vi "Check Transfer.vi"(8 "error in":errorcluster, 10 "TransferOperationResult":refnum<k24>, 11 "FileTransfer in":refnum<class "FileTransfer.lvclass">) -> (0 "error out":errorcluster, 3 "FileTransfer out":refnum<class "FileTransfer.lvclass">)   [LabVIEW 2015, in "WinSCP.lvlib" / "FileTransfer.lvclass"]
uses:
  FileTransfer.lvclass
  C:/Program Files (x86)/WinSCP/WinSCPnet.dll
  Program Files (x86)/WinSCP/WinSCPnet.dll
panel:
  out "Array 3":cluster{"Message":string, "Source":string}[](array[cluster])
  out "Array 2":T1(array[cluster])
  out "IsSuccess":bool
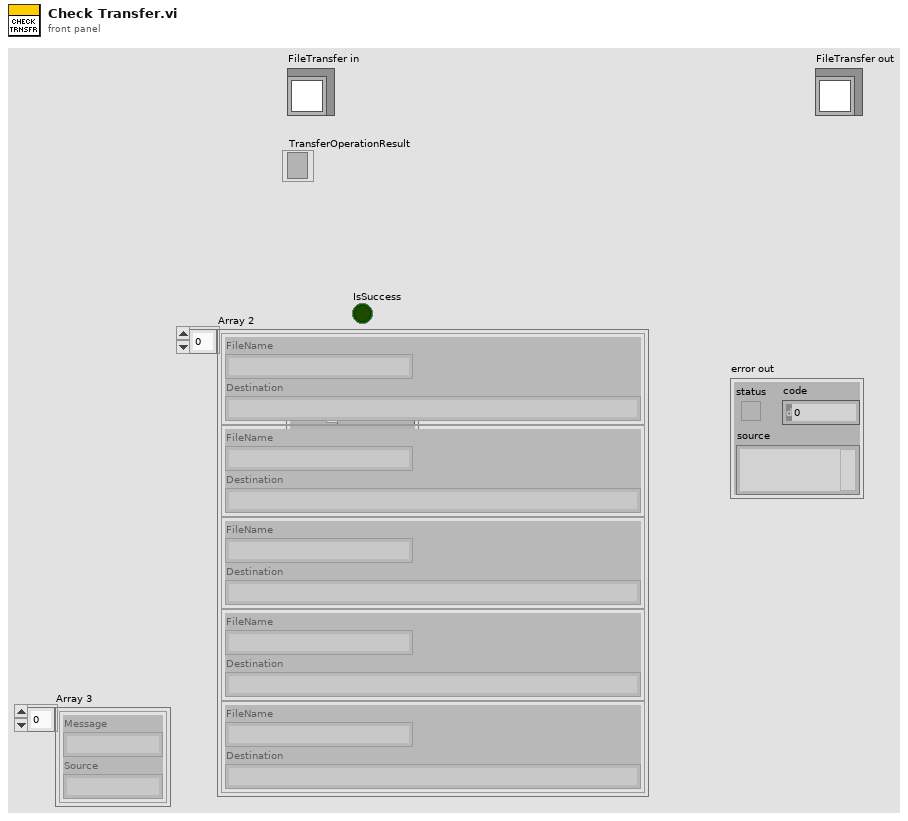
[diagram p1: front panel]
types:
  T1 = cluster{"FileName":string, "Destination":string}[]
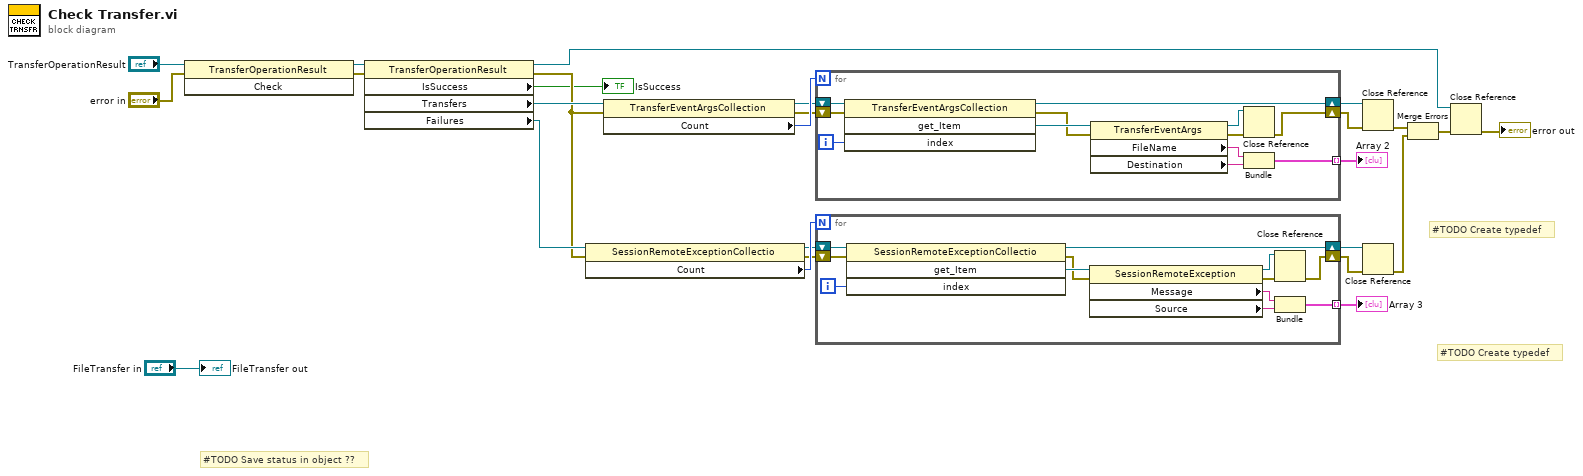
[diagram p0: block diagram]
diagram:
  # "#TODO Save status in object ??"
  # "#TODO Create typedef"
  # "#TODO Create typedef"
  n1 = invoke class="TransferOperationResult" method="Check"(reference="TransferOperationResult", error in="error in") -> (reference out=w25:refnum<k24>, error out=w8:errorcluster)  [unwired: 1 in, 1 out]
  n2 = property class="TransferOperationResult"(reference=w25, error in=w8) -> (reference out=w19:refnum<k24>, error out=w7:errorcluster, "IsSuccess"=→"IsSuccess":bool, "Transfers"=w24:refnum<k24>, "Failures"=w18:refnum<k24>)
  n3 = property class="SessionRemoteExceptionCollectio"(reference=w18, error in=w7) -> (reference out=w16:refnum<k24>, error out=w3:errorcluster, "Count"=w17:i32)
  n4 = property class="TransferEventArgsCollection"(reference=w24, error in=w7) -> (reference out=w22:refnum<k24>, error out=w5:errorcluster, "Count"=w23:i32)
  n5 = for {
    N: w23 -> [_]
    shift-right: [w33] -> w20
    shift-left: w22 -> [w38]
    tunnel: [w32] -> w21 mode=indexing
    shift-right: [w27] -> w4
    shift-left: w5 -> [w29]
    i -> [w37]
    n6 = invoke class="TransferEventArgsCollection" method="get_Item"(reference=w38, error in=w29, "index"=w37) -> (reference out=w33:refnum<k24>, error out=w28:errorcluster, "get_Item"=w36:refnum<k24>)  [unwired: 1 in, 1 out]
    n7 = property class="TransferEventArgs"(reference=w36, error in=w28) -> (reference out=w30:refnum<k24>, error out=w31:errorcluster, "FileName"=w35:string, "Destination"=w34:string)
    n8 = Close Reference(reference=w30, error in (no error)=w31) -> (error out=w27:errorcluster)
    n9 = Bundle("FileName"=w35, "Destination"=w34) -> (w32:cluster{"FileName":string, "Destination":string})  [unwired: 1 in]
  }
  "Array 2" <- w21
  n10 = for {
    N: w17 -> [_]
    shift-right: [w45] -> w14
    shift-left: w16 -> [w50]
    tunnel: [w44] -> w15 mode=indexing
    shift-right: [w39] -> w2
    shift-left: w3 -> [w41]
    i -> [w49]
    n11 = invoke class="SessionRemoteExceptionCollectio" method="get_Item"(reference=w50, error in=w41, "index"=w49) -> (reference out=w45:refnum<k24>, error out=w40:errorcluster, "get_Item"=w48:refnum<k24>)  [unwired: 1 in, 1 out]
    n12 = property class="SessionRemoteException"(reference=w48, error in=w40) -> (reference out=w42:refnum<k24>, error out=w43:errorcluster, "Message"=w47:string, "Source"=w46:string)
    n13 = Close Reference(reference=w42, error in (no error)=w43) -> (error out=w39:errorcluster)
    n14 = Bundle("Message"=w47, "Source"=w46) -> (w44:cluster{"Message":string, "Source":string})  [unwired: 1 in]
  }
  "Array 3" <- w15
  n15 = Close Reference(reference=w20, error in (no error)=w4) -> (error out=w13:errorcluster)
  n16 = Close Reference(reference=w14, error in (no error)=w2) -> (error out=w12:errorcluster)
  n17 = Merge Errors(w13, w12) -> (w11:errorcluster)
  n18 = Close Reference(reference=w19, error in (no error)=w11) -> (error out=→"error out":errorcluster)
  "FileTransfer out" <- "FileTransfer in"
